vi "模拟量设置窗口.vi"() -> ()   [LabVIEW 2016, in "环境动力监测库.lvlib"]
panel:
  out "AD7 工程量":dbl
  out "AD6 工程量":dbl
  out "AD7":dbl
  out "AD6":dbl
  in  "线性关系-通道 8":cluster{"X0":dbl, "X1":dbl, "Y0":dbl, "Y1":dbl} caption="线性关系-通道7"
  in  "线性关系-通道 7":cluster{"X0":dbl, "X1":dbl, "Y0":dbl, "Y1":dbl} caption="线性关系-通道6"
  out "AD5 工程量":dbl
  out "AD4 工程量":dbl
  out "AD3 工程量":dbl
  out "AD2 工程量":dbl
  out "AD1 工程量":dbl
  out "AD0 工程量":dbl
  in  "关闭":bool
  out "AD5":dbl
  out "AD4":dbl
  out "AD3":dbl
  out "AD2":dbl
  out "AD1":dbl
  out "AD0":dbl
  in  "线性关系-通道 6":cluster{"X0":dbl, "X1":dbl, "Y0":dbl, "Y1":dbl} caption="线性关系-通道5"
  in  "线性关系-通道 5":cluster{"X0":dbl, "X1":dbl, "Y0":dbl, "Y1":dbl} caption="线性关系-通道4"
  in  "线性关系-通道 4":cluster{"X0":dbl, "X1":dbl, "Y0":dbl, "Y1":dbl} caption="线性关系-通道3"
  in  "线性关系-通道 3":cluster{"X0":dbl, "X1":dbl, "Y0":dbl, "Y1":dbl} caption="线性关系-通道2"
  in  "线性关系-通道 2":cluster{"X0":dbl, "X1":dbl, "Y0":dbl, "Y1":dbl} caption="线性关系-通道1"
  in  "线性关系-通道":cluster{"X0":dbl, "X1":dbl, "Y0":dbl, "Y1":dbl} caption="线性关系-通道0"
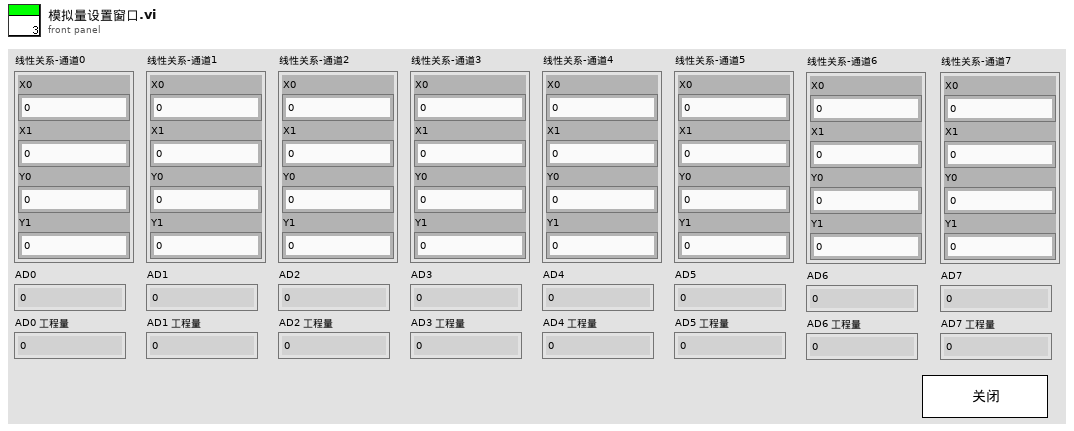
[diagram p1: front panel]
types:
  T1 = cluster{"AD0":dbl, "AD1":dbl, "AD1":dbl, "AD3":dbl, "AD4":dbl, "AD5":dbl, "AD6":dbl, "AD7":dbl}
  T2 = cluster{"AD0":dbl, "AD1":dbl, "AD2":dbl, "AD3":dbl, "AD4":dbl, "AD5":dbl, "AD6":dbl, "AD7":dbl}
  T3 = cluster{"X0":dbl, "X1":dbl, "Y0":dbl, "Y1":dbl}[]
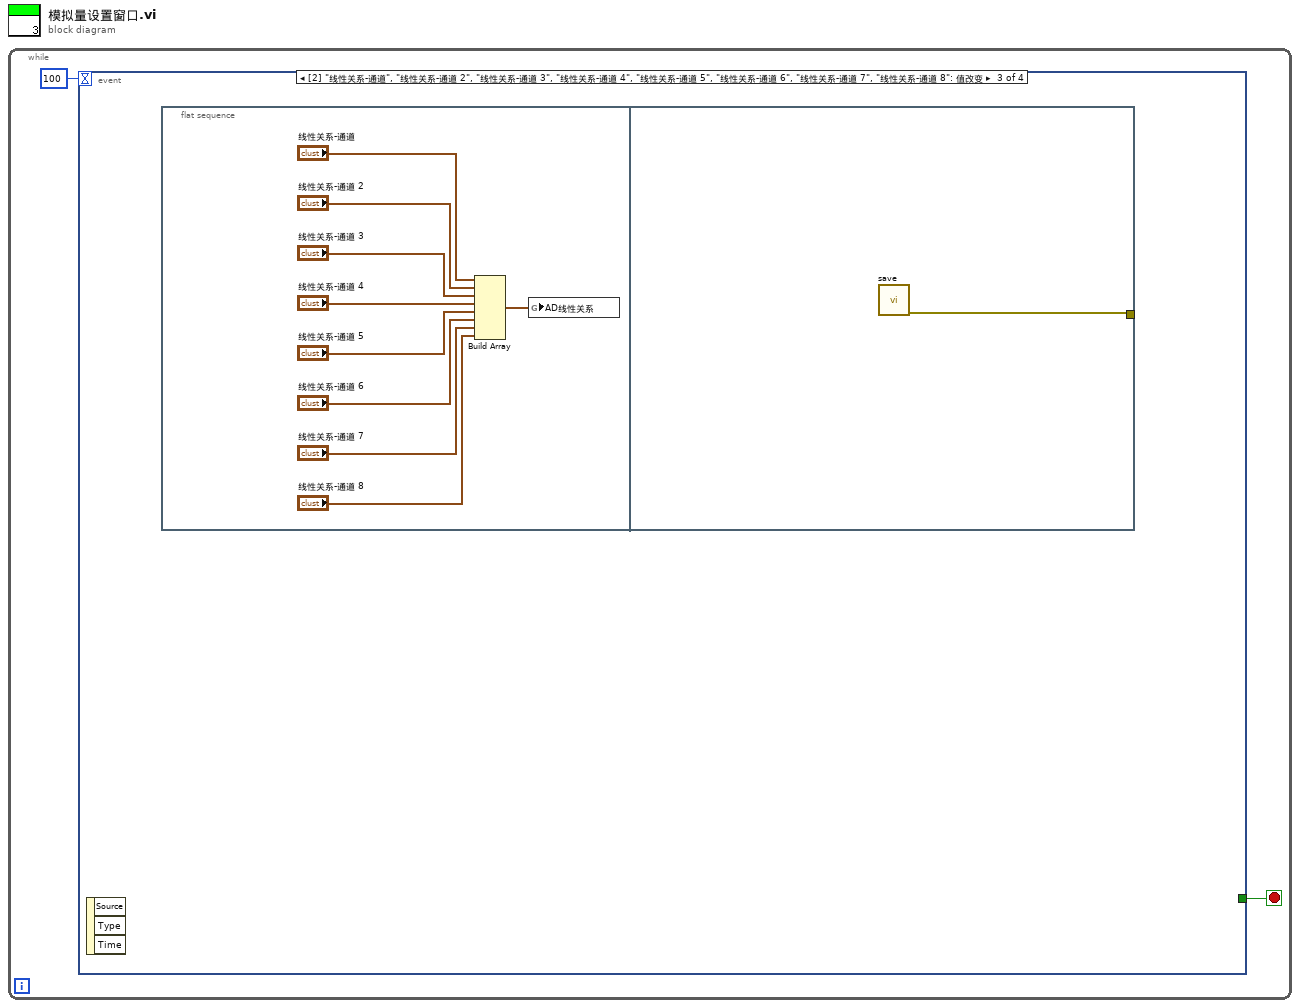
[diagram p0: block diagram]
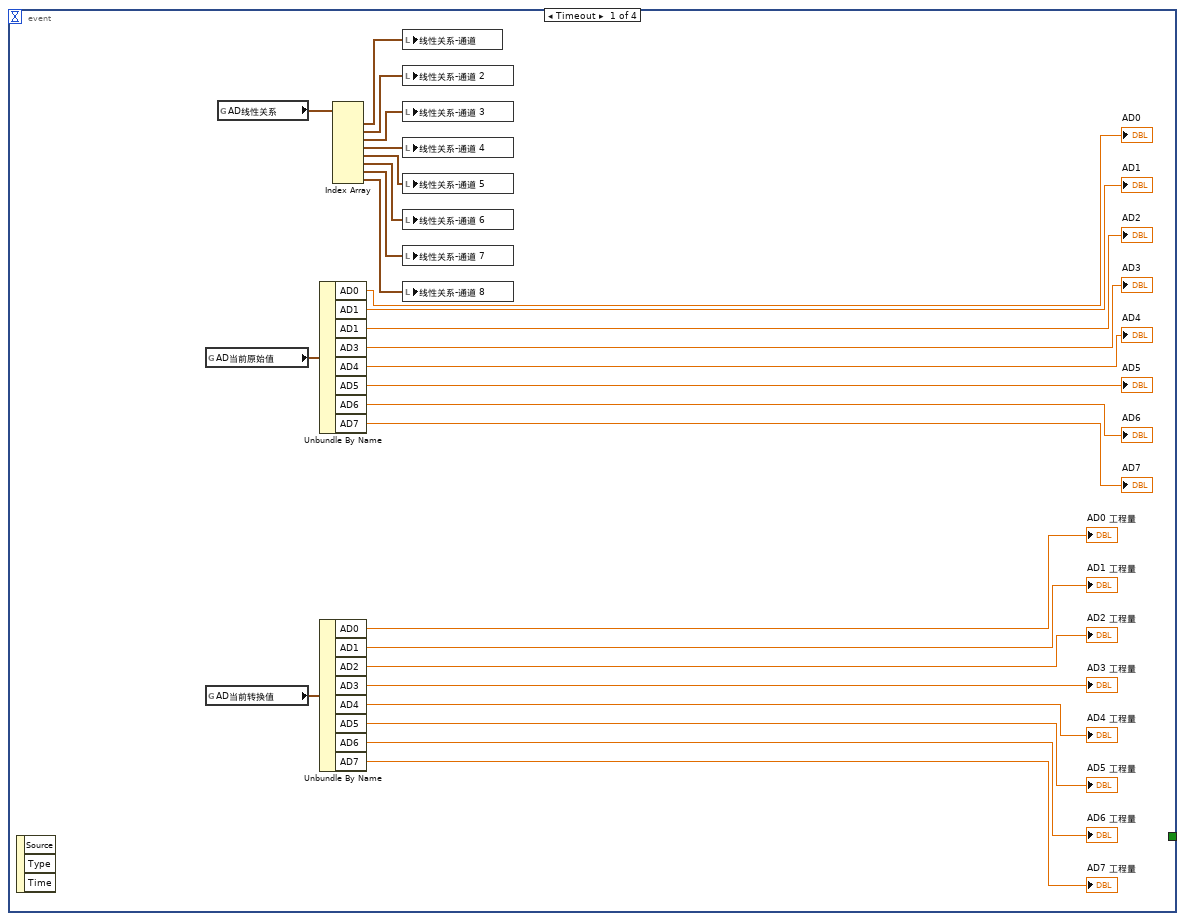
[diagram p2: hidden frame]
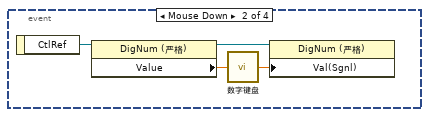
[diagram p3: hidden frame]
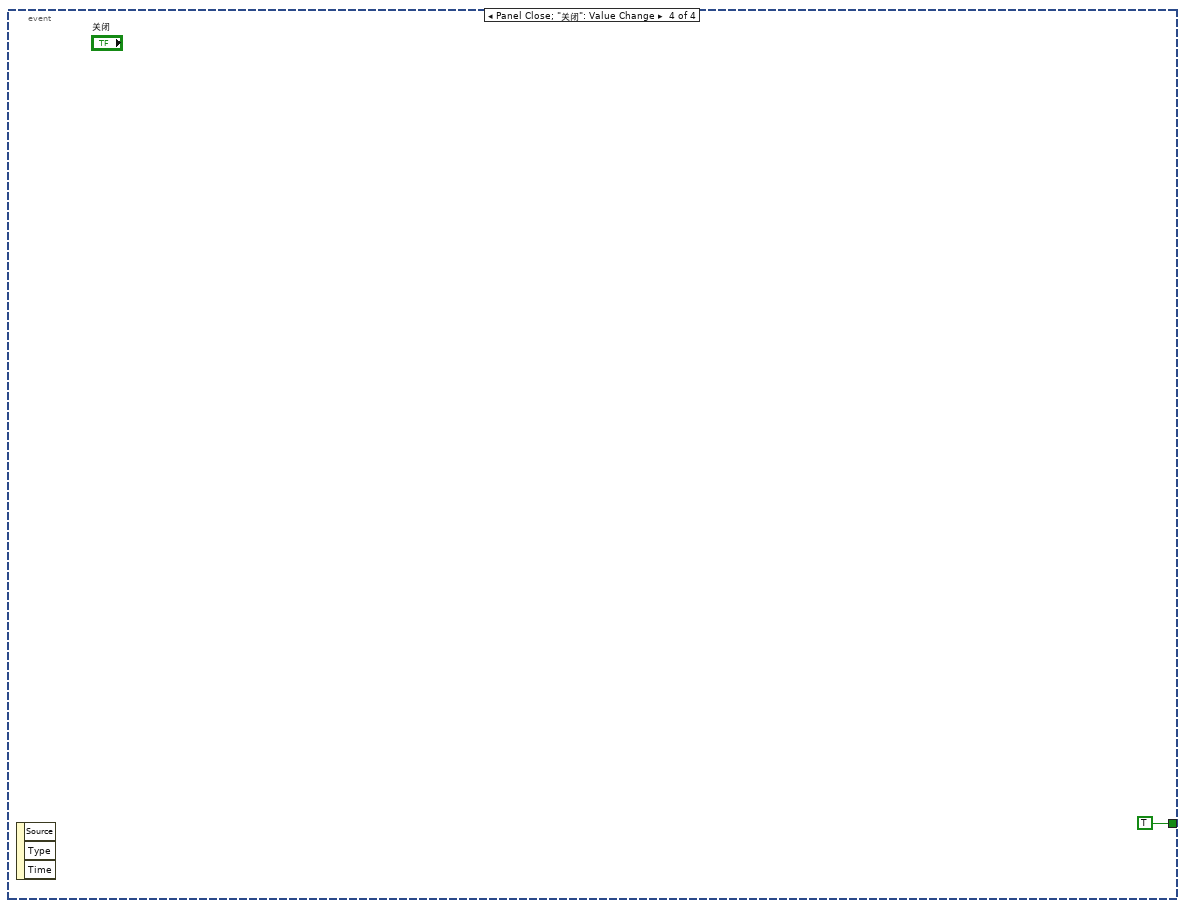
[diagram p4: hidden frame]
diagram:
  n1 = while {
    stop <- w2 stop-if-true
    n2 = event shown="[2] \"线性关系-通道\", \"线性关系-通道 2\", \"线性关系-通道 3\", \"线性关系-通道 4\", \"线性关系-通道 5\", \"线性关系-通道 6\", \"线性关系-通道 7\", \"线性关系-通道 8\": 值改变" {
      selector: _ -> [_ _ _ _]
      dyn-events: _ -> [_ _ _ _]
      timeout: 100 -> [_ _ _ _]
      tunnel: [_ _ _ TRUE] -> w2
      event Timeout {
        n3 = event-data() -> ()  [unwired: 1 in, 3 out]
        n4 = global read "断电保存全局变量.vi" "AD当前原始值"() -> (w11:T1)
        n5 = global read "断电保存全局变量.vi" "AD当前转换值"() -> (w10:T2)
        n6 = global read "断电保存全局变量.vi" "AD线性关系"() -> (w9:T3)
        n7 = Unbundle By Name(w11) -> ("AD0"=→"AD0":dbl, "AD1"=→"AD1":dbl, "AD1"=→"AD2":dbl, "AD3"=→"AD3":dbl, "AD4"=→"AD4":dbl, "AD5"=→"AD5":dbl, "AD6"=→"AD6":dbl, "AD7"=→"AD7":dbl)
        n8 = Unbundle By Name(w10) -> ("AD0"=→"AD0 工程量":dbl, "AD1"=→"AD1 工程量":dbl, "AD2"=→"AD2 工程量":dbl, "AD3"=→"AD3 工程量":dbl, "AD4"=→"AD4 工程量":dbl, "AD5"=→"AD5 工程量":dbl, "AD6"=→"AD6 工程量":dbl, "AD7"=→"AD7 工程量":dbl)
        n9 = Index Array(array=w9) -> (element #1=w23:cluster{"X0":dbl, "X1":dbl, "Y0":dbl, "Y1":dbl}, element #2=w22:cluster{"X0":dbl, "X1":dbl, "Y0":dbl, "Y1":dbl}, element #3=w21:cluster{"X0":dbl, "X1":dbl, "Y0":dbl, "Y1":dbl}, element #4=w20:cluster{"X0":dbl, "X1":dbl, "Y0":dbl, "Y1":dbl}, element #5=w19:cluster{"X0":dbl, "X1":dbl, "Y0":dbl, "Y1":dbl}, element #6=w18:cluster{"X0":dbl, "X1":dbl, "Y0":dbl, "Y1":dbl}, element #7=w4:cluster{"X0":dbl, "X1":dbl, "Y0":dbl, "Y1":dbl}, element #8=w3:cluster{"X0":dbl, "X1":dbl, "Y0":dbl, "Y1":dbl})  [unwired: 8 in]
        n10 = local write "线性关系-通道"(w23) -> ()
        n11 = local write "线性关系-通道 2"(w22) -> ()
        n12 = local write "线性关系-通道 3"(w21) -> ()
        n13 = local write "线性关系-通道 4"(w20) -> ()
        n14 = local write "线性关系-通道 5"(w19) -> ()
        n15 = local write "线性关系-通道 6"(w18) -> ()
        n16 = local write "线性关系-通道 7"(w4) -> ()
        n17 = local write "线性关系-通道 8"(w3) -> ()
      }
      event "线性关系-通道.X0", "线性关系-通道.X1", "线性关系-通道.Y0", "线性关系-通道.Y1", "线性关系-通道 2.X0", "线性关系-通道 2.X1", "线性关系-通道 2.Y0", "线性关系-通道 2.Y1", "线性关系-通道 3.X0", "线性关系-通道 3.X1", "线性关系-通道 3.Y0", "线性关系-通道 3.Y1", "线性关系-通道 4.X0", "线性关系-通道 4.X1", "线性关系-通道 4.Y0", "线性关系-通道 4.Y1", "线性关系-通道 5.X0", "线性关系-通道 5.X1", "线性关系-通道 5.Y0", "线性关系-通道 5.Y1", "线性关系-通道 6.X0", "线性关系-通道 6.X1", "线性关系-通道 6.Y0", "线性关系-通道 6.Y1", "线性关系-通道 7.X0", "线性关系-通道 7.X1", "线性关系-通道 7.Y0", "线性关系-通道 7.Y1", "线性关系-通道 8.X0", "线性关系-通道 8.X1", "线性关系-通道 8.Y0", "线性关系-通道 8.Y1": Mouse Down {
        n18 = event-data() -> ("CtlRef"=w33:refnum<vi>)  [unwired: 1 in]
        n19 = property class="DigNum (严格)"(reference=w33) -> (reference out=w31:refnum<vi>, "Value"=w32:dbl)  [unwired: 1 in, 1 out]
        n20 = call "数字键盘.vi"("OldNumber"=w32) -> ("NewNumber"=w30:sgl)
        n21 = property class="DigNum (严格)"(reference=w31, "Val(Sgnl)"=w30) -> ()  [unwired: 1 in, 2 out]
      }
      event "线性关系-通道", "线性关系-通道 2", "线性关系-通道 3", "线性关系-通道 4", "线性关系-通道 5", "线性关系-通道 6", "线性关系-通道 7", "线性关系-通道 8": Value Change {
        n22 = event-data() -> ()  [unwired: 1 in, 3 out]
        n23 = flat-sequence {
          tunnel: [w43] -> _
          frame #0 {
            n24 = Build Array("线性关系-通道", "线性关系-通道 2", "线性关系-通道 3", "线性关系-通道 4", "线性关系-通道 5", "线性关系-通道 6", "线性关系-通道 7", "线性关系-通道 8") -> (w36:T3)
            n25 = global write "断电保存全局变量.vi" "AD线性关系"(w36) -> ()
          }
          frame #1 {
            n26 = call "save.vi"() -> ("error out"=w43:errorcluster)  [unwired: 11 in]
          }
        }
      }
      event Panel Close; "关闭": Value Change {
        n27 = event-data() -> ()  [unwired: 1 in, 3 out]
      }
    }
  }
